vi "Close File.vi"(8 "error in":errorcluster) -> (0 "error out":errorcluster)   [LabVIEW 2018, in "Support Library.lvlib" / "Command Logging.lvlib"]
uses:
  Command Logging.lvlib
  File Path.ctl
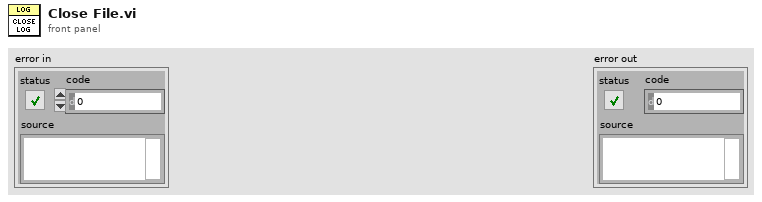
[diagram p1: front panel]
types:
  T1 = typedef "Support Library.lvlib/Command Logging.lvlib/File Path.ctl" = refnum<file>
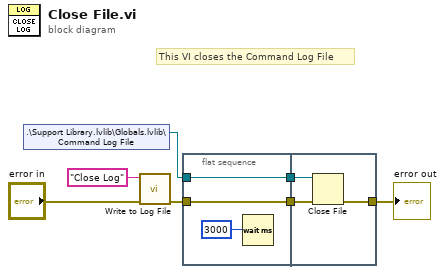
[diagram p0: block diagram]
diagram:
  # "This VI closes the Command Log File"
  n1 = shared-variable ".\\Support Library.lvlib\\Globals.lvlib\\Command Log File"() -> (w3:T1)  [unwired: 1 in, 1 out]
  n2 = call "Write to Log File.vi"("error in"="error in", "text"="Close Log") -> ("error out"=w5:errorcluster)  [unwired: 9 in]
  n3 = flat-sequence {
    tunnel: w3 -> [w9]
    tunnel: w5 -> [w10]
    tunnel: [w10] -> w2
    tunnel: [w9] -> w1
    tunnel: [w13] -> w7
    tunnel: w2 -> [w12]
    tunnel: w1 -> [w11]
    frame #0 {
      n4 = Wait (ms)(milliseconds to wait=u32 3000) -> ()  [unwired: 1 out]
    }
    frame #1 {
      n5 = Close File(refnum=w11, error in=w12) -> (error out=w13:errorcluster)  [unwired: 1 out]
    }
  }
  "error out" <- w7
